vi "PSVH_Bool String Check.vi"(10 "Bool Str":string) -> (1 "Boolean":bool, 2 "Bool?":bool)   [LabVIEW 2016]
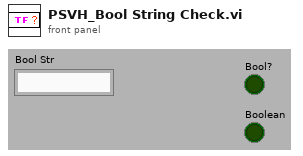
[diagram p1: front panel]
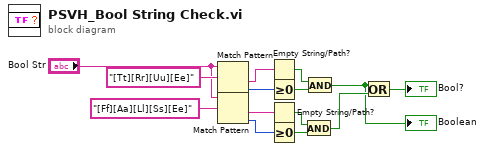
[diagram p0: block diagram]
diagram:
  n1 = Match Pattern(string="Bool Str", regular expression="[Tt][Rr][Uu][Ee]") -> (after substring=w10:string, offset past match=w11:i32)  [unwired: 1 in, 2 out]
  n2 = Match Pattern(string="Bool Str", regular expression="[Ff][Aa][Ll][Ss][Ee]") -> (after substring=w8:string, offset past match=w9:i32)  [unwired: 1 in, 2 out]
  n3 = Empty String/Path?(string/path=w10) -> (empty?=w5:bool)
  n4 = Greater Or Equal To 0?(x=w11) -> (x >= 0?=w4:bool)
  n5 = Empty String/Path?(string/path=w8) -> (empty?=w6:bool)
  n6 = Greater Or Equal To 0?(x=w9) -> (x >= 0?=w7:bool)
  n7 = And(x=w6, y=w7) -> (x .and. y?=w3:bool)
  n8 = And(x=w5, y=w4) -> (x .and. y?=w1:bool)
  "Boolean" <- w1
  n9 = Or(x=w1, y=w3) -> (x .or. y?=→"Bool?":bool)
